vi "Chanotch.vi"(0 "Signal":dbl[](array[numeric]), 1 "Freq":dbl[](array[numeric])) -> (2 "Chanotched Signal":dbl[](array[numeric]))   [LabVIEW 2009]
uses:
  <vilib>/Analysis/2dsp.llb/Inverse Complex FFT.vi
  <vilib>/Analysis/2dsp.llb/Real FFT.vi
  <vilib>/Analysis/NI_AALPro.lvlib
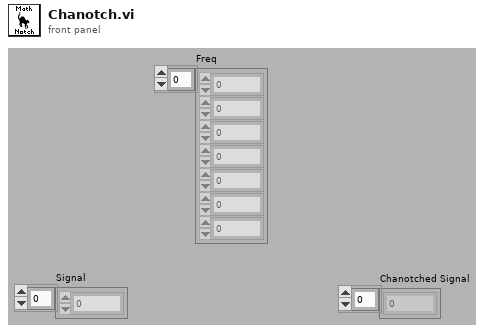
[diagram p1: front panel]
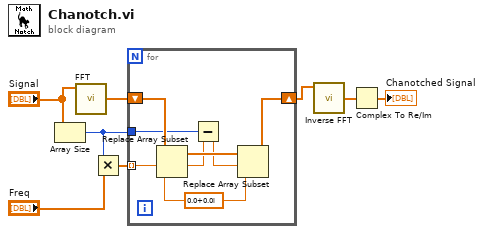
[diagram p0: block diagram]
diagram:
  n1 = Array Size(array="Signal") -> (size(s)=w1:i32)
  n2 = call-poly <vilib>:"FFT.vi"("X"="Signal") -> ("FFT {X}"=w5:cdb[])  [unwired: 9 in, 1 out]
  n3 = Multiply(x=w1, y="Freq") -> (x*y=w3:dbl[])
  n4 = for {
    shift-right: [w12] -> w4
    shift-left: w5 -> [w15]
    tunnel: w3 -> [w11] mode=indexing
    tunnel: w1 -> [w10]
    w14 = cdb 0.0+0.0i ("nouvel élt/sous-tableau")
    n5 = Replace Array Subset(array=w15, new element=w14, index=w11) -> (w13:cdb[])
    n6 = Subtract(x=w10, y=w11) -> (x-y=w9:dbl)
    n7 = Replace Array Subset(array=w13, new element=w14, index=w9) -> (w12:cdb[])
  }
  n8 = call-poly <vilib>:"Inverse FFT.vi"("FFT {X}"=w4) -> ("X"=w7:cdb[])  [unwired: 9 in, 1 out]
  n9 = Complex To Re/Im(x + iy=w7) -> (x=→"Chanotched Signal":dbl[])  [unwired: 1 out]
